vi "LogControlData.vi"(8 "Fault":bool, 9 "RobotControl":cluster{"VlProfile":i16[], "VrProfile":i16[]}, 10 "StateParams":T1={"FPGARef"=refnum, "Sync"=FALSE, "FullState"=[], "ControlParams"={"Kx"=30.0, "Ky"=1.0, "Kt"=50.0, "d"=0.07, "Ks"=80.0, "MinV"=0.0, "MaxV"=1000.0, "Ka"=0.07}}, 11 "ControlStream":refnum<file>) -> ()   [LabVIEW 2011]
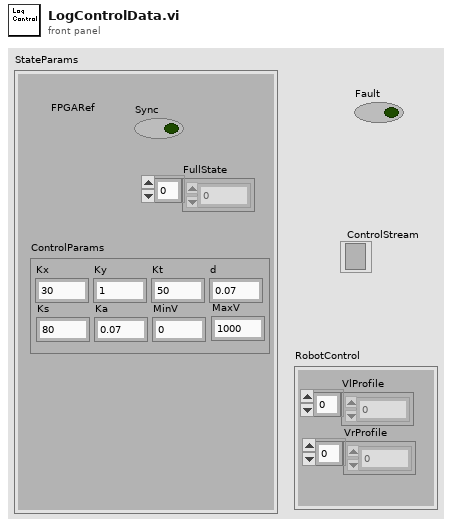
[diagram p1: front panel]
types:
  T1 = cluster{"FPGARef":refnum<k20>, "Sync":bool, "FullState":dbl[], "ControlParams":cluster{"Kx":dbl, "Ky":dbl, "Kt":dbl, "d":dbl, "Ks":dbl, "MinV":dbl, "MaxV":dbl, "Ka":dbl}}
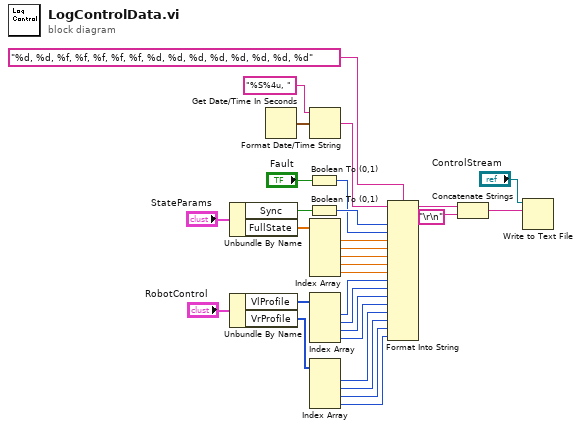
[diagram p0: block diagram]
diagram:
  n1 = Unbundle By Name("StateParams") -> ("Sync"=w19:bool, "FullState"=w21:dbl[])
  n2 = Unbundle By Name("RobotControl") -> ("VlProfile"=w17:i16[], "VrProfile"=w16:i16[])
  n3 = Get Date/Time In Seconds() -> (seconds since 1Jan1904=w25:timestamp)
  n4 = Boolean To (0,1)(Boolean="Fault") -> (0, 1=w15:i16)
  n5 = Boolean To (0,1)(Boolean=w19) -> (0, 1=w18:i16)
  n6 = Format Date/Time String(time format string (%c)="%S%4u, " ("format string"), seconds (now)=w25) -> (date/time string=w27:string)  [unwired: 1 in]
  n7 = Index Array(array=w21) -> (element #1=w13:dbl, element #2=w12:dbl, element #3=w11:dbl, element #4=w10:dbl, element #5=w9:dbl)  [unwired: 5 in]
  n8 = Index Array(array=w17) -> (element #1=w8:i16, element #2=w7:i16, element #3=w6:i16, element #4=w5:i16)  [unwired: 4 in]
  n9 = Index Array(array=w16) -> (element #1=w4:i16, element #2=w3:i16, element #3=w2:i16, element #4=w1:i16)  [unwired: 4 in]
  n10 = Format Into String(format string="%d, %d, %f, %f, %f, %f, %f, %d, %d, %d, %d, %d, %d, %d, %d", initial string=w27, w18, w15, w13, w12, w11, w10, w9, w8, w7, w6, w5, w4, w3, w2, w1) -> (resulting string=w28:string)  [unwired: 1 in, 1 out]
  n11 = Concatenate Strings(w28, "\r\n") -> (w30:string)
  n12 = Write to Text File(file (use dialog)="ControlStream", text=w30) -> ()  [unwired: 2 in, 3 out]
